vi "Read Multiple Digital Channels.vi"(8 "error in (no error)":errorcluster, 10 "Digital Pin":T2(array[ring]), 11 "VISA resource name":refnum<visa-resource-name>) -> (0 "error out":errorcluster, 2 "Array":bool[](array[boolean]), 3 "VISA resource name out":refnum<visa-resource-name>)   [LabVIEW 2020, in "BDAQ-6104.lvlib"]
uses:
  <instrlib>/BDAQ-6104/BDAQ-6104.lvlib
panel:
  out "Digital Pin Number":T1(ring)
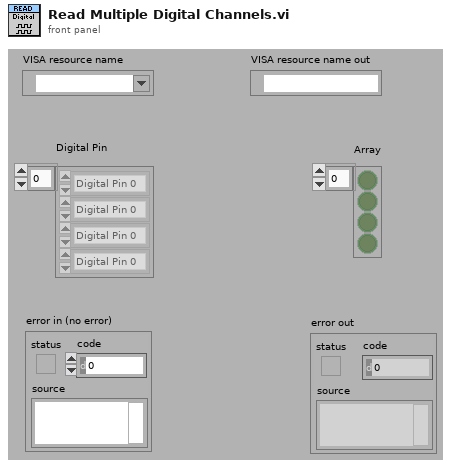
[diagram p1: front panel]
types:
  T1 = enum16{"Digital Pin 0", "Digital Pin 1", "Digital Pin 2", "Digital Pin 3"}
  T2 = enum16{"Digital Pin 0", "Digital Pin 1", "Digital Pin 2", "Digital Pin 3"}[]
  T3 = cluster{"DIO0":bool, "DIO1":bool, "DIO2":bool, "DIO3":bool}
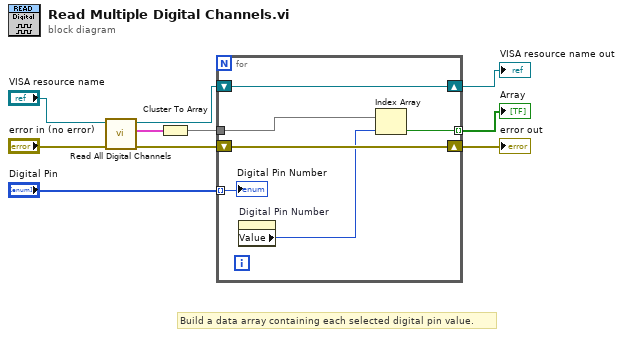
[diagram p0: block diagram]
diagram:
  # "Build a data array containing each selected digital pin value."
  n1 = call <instrlib>:"Read All Digital Channels.vi"("error in (no error)"="error in (no error)", "VISA resource name"="VISA resource name") -> ("error out"=w5:errorcluster, "Digital Outputs"=w2:T3, "VISA resource name out"=w7:refnum<visa-resource-name>)  [unwired: 6 in]
  n2 = Cluster To Array(cluster=w2) -> (array=w1:bool[])
  n3 = for {
    tunnel: "Digital Pin" -> [w13] mode=indexing
    shift-right: [w15] -> w4
    shift-left: w5 -> [w15]
    tunnel: [w14] -> w3 mode=indexing
    shift-right: [w16] -> w6
    shift-left: w7 -> [w16]
    tunnel: w1 -> [w11]
    n4 = property on="Digital Pin Number" class="Enum (strict)"() -> ("Value"=w12:T1)  [unwired: 2 in, 2 out]
    n5 = Index Array(array=w11, index=w12) -> (element=w14:bool)
    "Digital Pin Number" <- w13
  }
  "VISA resource name out" <- w6
  "error out" <- w4
  "Array" <- w3
